vi "writeDataFile.vi"(8 "error in (no error)":errorcluster, 10 "WriteDataFileInput":T1, 11 "CSVTestLog in":refnum<class "CSVTestLog.lvclass">) -> (0 "error out":errorcluster, 2 "Relative Path":string, 3 "CSVTestLog out":refnum<class "CSVTestLog.lvclass">)   [LabVIEW 2015, in "CSVTestLog.lvclass"]
uses:
  CSVTestLog.lvclass
  Typedefs/WriteDataFileInput.ctl
  Typedefs/TestScenarioTypes.ctl
  Typedefs/ILCBTTypedefs.lvlib
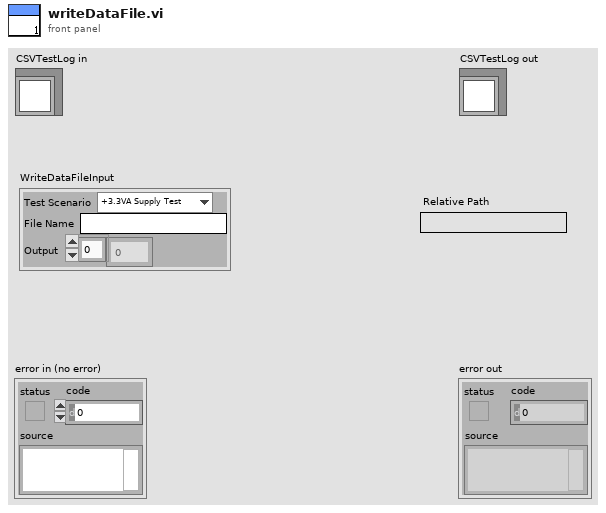
[diagram p1: front panel]
types:
  T1 = typedef "ILCBTTypedefs.lvlib/WriteDataFileInput.ctl" = cluster{"Test Scenario":T2, "File Name":string, "Output":dbl[]}
  T2 = typedef "ILCBTTypedefs.lvlib/TestScenarioTypes.ctl" = enum16{"+3.3VA Supply Test", "+3.3VD Supply Test", "+5VA Supply Test", "+5VD Supply Test"}
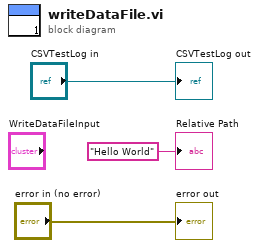
[diagram p0: block diagram]
diagram:
  "error out" <- "error in (no error)"
  "CSVTestLog out" <- "CSVTestLog in"
  "Relative Path" <- "Hello World" ("Relative Path")
